vi "Fast Set Item Property (Dependent Node Pointer) FuncGlobal.vi"(5 "Action":enum16{"Open or Add", "Close Ref"}(ring), 8 "error in (no error)":errorcluster, 9 "Dependent Node Ref":T1=18446744073709551615 format="%.0x", 10 "Property Name":string, 11 "Item Ref in":T1 format="%.0x") -> (0 "error out":errorcluster, 3 "Item Ref out":T1 format="%.0x", 4 "Replaced":bool)   [LabVIEW 2011]
doc: "Sets a <B>Property Name</B> and <B>Value</B> for an item. If the <B>Property Name</B> you specify already exists, NI VeriStand overwrites the property."
uses:
  <vilib>/NI Veristand/Custom Device API/Custom Device Item Ref.ctl
  <vilib>/NI Veristand/Custom Device API/Custom Device API.lvlib
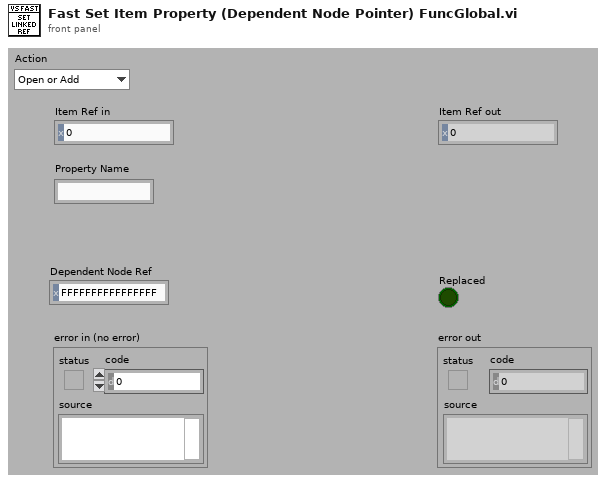
[diagram p1: front panel]
types:
  T1 = typedef "Custom Device API.lvlib/Custom Device Item Ref.ctl" = u64
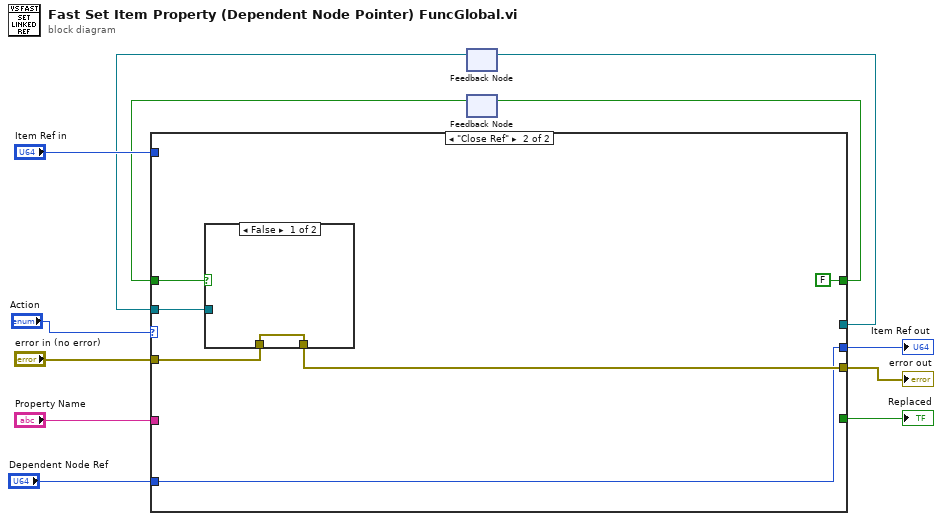
[diagram p0: block diagram]
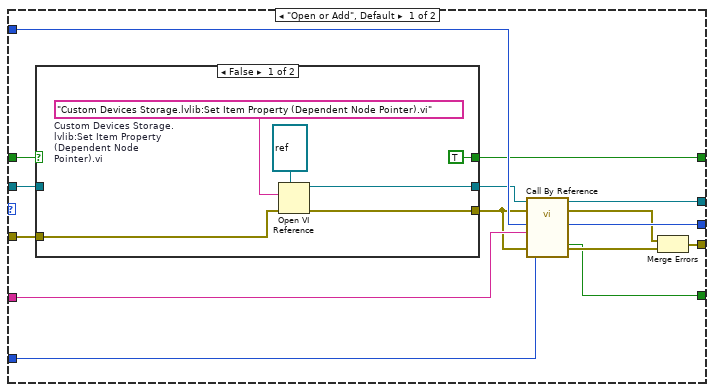
[diagram p2: hidden frame]
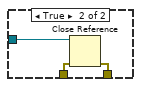
[diagram p4: hidden frame]
diagram:
  n1 = feedback #1() -> (w2:refnum<vi>)  [unwired: 1 in]
  n2 = feedback #2() -> (w3:bool)  [unwired: 1 in]
  n3 = case shown="\"Close Ref\"" "Action" {
    tunnel: "error in (no error)" -> [w26 w40]
    tunnel: "Item Ref in" -> [w25 _]
    tunnel: [w24 w37] -> w10
    tunnel: [w23 w39] -> w9
    tunnel: "Property Name" -> [w22 _]
    tunnel: [w21 _] -> w7
    tunnel: "Dependent Node Ref" -> [w20 w37]
    tunnel: [w17 _] -> w5
    tunnel: [w15 FALSE] -> w4
    tunnel: w3 -> [w14 w42]
    tunnel: w2 -> [w13 w41]
    frame "Open or Add", Default {
      n4 = case shown="False" w14 {
        selector: w14 -> [_ w36]
        tunnel: w26 -> [w31 w34]
        tunnel: [w30 w35] -> w19
        tunnel: [w29 w34] -> w18
        tunnel: [TRUE w36] -> w15
        tunnel: w13 -> [_ w35]
        frame False {
          w33 = "Custom Devices Storage.lvlib:Set Item Property (Dependent Node Pointer).vi"  # Custom Devices Storage.lvlib:Set Item Property (Dependent Node Pointer).vi
          n5 = Open VI Reference(type specifier VI Refnum (for type only)=refnum<vi> refnum, vi path=w33, error in (no error)=w31) -> (vi reference=w30:refnum<vi>, error out=w29:errorcluster)  [unwired: 1 in, 2 out]
        }
        frame True {
        }
      }
      n6 = call-by-ref "?"(reference=w19, error in=w18, 8:"error in (no error)"=w18, "Dependent Node"=w20, "Property Name"=w22, "Item Ref in"=w25) -> (reference out=w17:refnum<vi>, error out=w16:errorcluster, 0:"error out"=w27:errorcluster, "Item Ref out"=w24:T1, "Replaced"=w21:bool)  [unwired: 5 in]
      n7 = Merge Errors(w16, w27) -> (w23:errorcluster)
    }
    frame "Close Ref" {
      n8 = case shown="False" w42 {
        tunnel: w41 -> [_ w46]
        tunnel: w40 -> [w43 w45]
        tunnel: [w43 w44] -> w39
        frame False {
        }
        frame True {
          n9 = Close Reference(reference=w46, error in (no error)=w45) -> (error out=w44:errorcluster)
        }
      }
    }
  }
  "Item Ref out" <- w10
  "error out" <- w9
  "Replaced" <- w7
  n10 = feedback-in #1(w5) -> ()
  n11 = feedback-in #2(w4) -> ()
